vi "INIT_events_SD.vi"(2 "bounds":T2, 3 "references":T1) -> (0 "main cluster":T3={"Kinetics"=[], "Spectrum"=[], "Experiments groups"=[], "GRAPH EXPERIMENTAL DATA"=[], "error out"={"status"=FALSE, "code"=0, "source"=""}, "group"=0, "exp selected"=0, "# exp"=0, "kinetics plot names"=[], "spectra plot names"=[], "FromToWave"={"FromWave"=0.0, "ToWave"=0.0}, "Laser shutter task"="", "Accelerator task"="", "Motor task"="", "GRAPH EXPERIMENTAL DATA ref"=refnum, "timedelays"=[0.0, 0.0, 0.0, 0.0, 0.0, 0.0, 0.0, 0.06019061100911815, 0.0521779104562645, 0.045231877429679615, 0.03921051490799832, 0.033990728811568754, 0.029465811603150715, 0.025543260876973825, 0.02214288834180205, 0.01919518054014414, 0.016639877791965713, 0.014424742312398925, 0.012504490320209958, 0.010839866306230088, 0.009396840537117498, 0.008145913389103785, 0.00706151229029317, 0.006121468943269439, 0.005306566140927374, 0.004600144911132549, 0.003987763959109073, 0.0034569044455719407, 0.00299671406541447, 0.0025977851951783253, 0.0022519625739982996, 0.00195217658646366, 0.0016922987392150965, 0.0014670163768006634, 0.0012717240756200802, 0.0011024294957352762, 0.0009556717658856477, 0.0008284507332614981, 0.0007181656316962257, 0.0006225619144775864, 0.0005396851648867825, 0.00046784114226338394, 0.0004055611468220084, 0.0003515719951773376, 0.00030476999279031153, 0.00026419837125694315, 0.00022902772919263772, 0.0001985390768670671, 0.0001721091379728629, 0.00014919760805372974, 0.00012933610911736794], "wavelengths"=[0.0, 0.0, 0.0, 0.0, 0.0, 0.0, 0.0, 0.06019061100911815, 0.0521779104562645, 0.045231877429679615, 0.03921051490799832, 0.033990728811568754, 0.029465811603150715, 0.025543260876973825, 0.02214288834180205, 0.01919518054014414, 0.016639877791965713, 0.014424742312398925, 0.012504490320209958, 0.010839866306230088, 0.009396840537117498, 0.008145913389103785, 0.00706151229029317, 0.006121468943269439, 0.005306566140927374, 0.004600144911132549, 0.003987763959109073, 0.0034569044455719407, 0.00299671406541447, 0.0025977851951783253, 0.0022519625739982996, 0.00195217658646366, 0.0016922987392150965, 0.0014670163768006634, 0.0012717240756200802, 0.0011024294957352762, 0.0009556717658856477, 0.0008284507332614981, 0.0007181656316962257, 0.0006225619144775864, 0.0005396851648867825, 0.00046784114226338394, 0.0004055611468220084, 0.0003515719951773376, 0.00030476999279031153, 0.00026419837125694315, 0.00022902772919263772, 0.0001985390768670671, 0.0001721091379728629, 0.00014919760805372974, 0.00012933610911736794], "Experiment"=refnum, "Commentaires exp"=refnum, "FromToDelay"={"FromDelay"=0.0, "ToDelay"=0.0}}, 1 "Controls":T4)   [LabVIEW 2015]
uses:
  controls/Controls.ctl
  Classes/Experiment.lvclass
  controls/control-cluster.ctl
  Classes/Experiments_group.lvclass
  globalVarSD.vi
types:
  T1 = cluster{"Commentaires exp":refnum<vi>, "GRAPH EXPERIMENTAL DATA":refnum<vi>, "Experiment":refnum<vi>}
  T2 = cluster{"From Time":dbl, "To Time":dbl, "From Wave":dbl, "To Wave":dbl}
  T3 = typedef "control-cluster.ctl" = cluster{"Kinetics":cluster{"timedelay":dbl[], dbl[]}[], "Spectrum":cluster{"Unités abscisse":dbl[], dbl[]}[], "Experiments groups":refnum<class "Experiments_group.lvclass">[], "GRAPH EXPERIMENTAL DATA":dbl[][], "error out":errorcluster, "group":i32, "exp selected":i32, "# exp":i32, "kinetics plot names":string[], "spectra plot names":string[], "FromToWave":cluster{"FromWave":dbl, "ToWave":dbl}, "Laser shutter task":refnum<k21>, "Accelerator task":refnum<k21>, "Motor task":refnum<k21>, "GRAPH EXPERIMENTAL DATA ref":refnum<vi>, "timedelays":dbl[], "wavelengths":dbl[], "Experiment":refnum<vi>, "Commentaires exp":refnum<vi>, "FromToDelay":cluster{"FromDelay":dbl, "ToDelay":dbl}}
  T4 = typedef "Controls.ctl" = cluster{"Update graphs of exp":refnum<user-event>, "Reglage event":refnum<user-event>, "Stop event":refnum<user-event>, "notifier mesure out":refnum<notifier>, "notifier reglage out":refnum<notifier>, "Measure finished":refnum<user-event>, "control registration ref":refnum<event-registration>, "redraw event":refnum<user-event>, "Measure event":refnum<user-event>, "Mes, Reg, Stop Registration ref":refnum<event-registration>, "Laser shutter task":refnum<k21>, "error out":errorcluster, "Motor task":refnum<k21>, "Accelerator task":refnum<k21>, "Faraday Cup task":refnum<k21>, "Protection":refnum<event-registration>, "heater Alarm task":refnum<k21>, "Relay key task":refnum<k21>}
  T5 = cluster{"Heater alaram task":refnum<k21>, "Laser shutter task":refnum<k21>, "Motor task":refnum<k21>, "Accelerator shutter task":refnum<k21>, "Relay key task":refnum<k21>, "Faraday cup task":refnum<k21>}
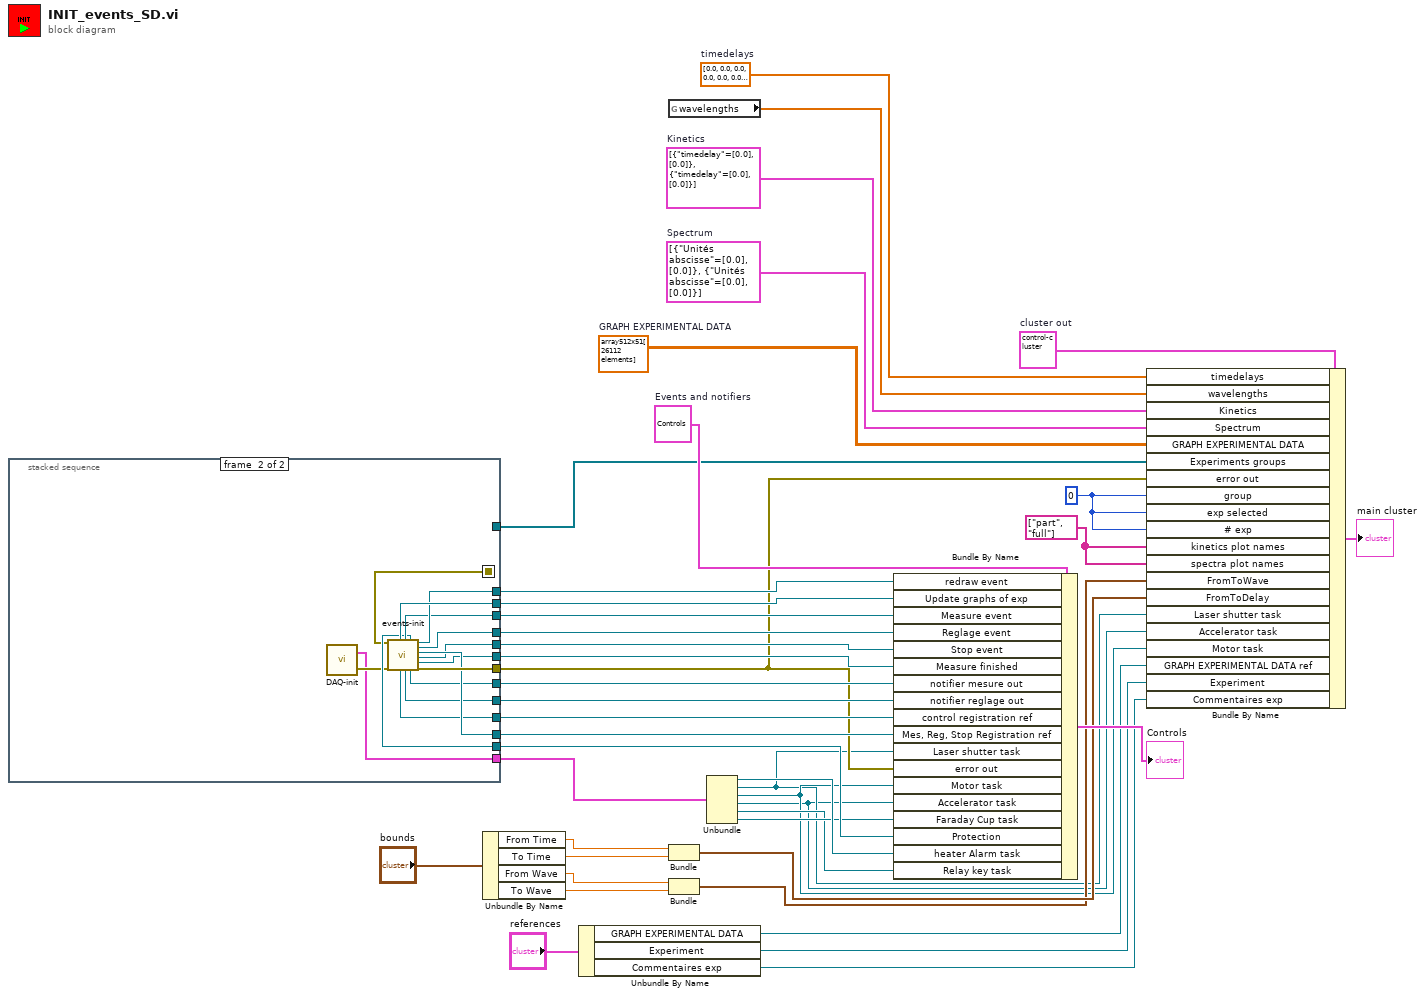
[diagram p0: block diagram]
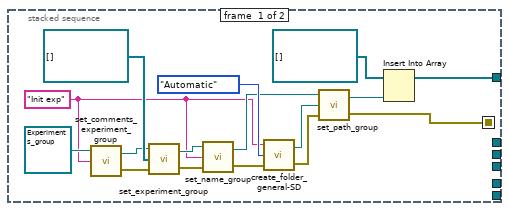
[diagram p2: hidden frame]
diagram:
  w18 = dbl[] [0.0, 0.0, 0.0, 0.0, 0.0, 0.0, 0.0, 0.06019061100911815, 0.0521779104562645, 0.045231877429679615, 0.03921051490799832, 0.033990728811568754, 0.029465811603150715, 0.025543260876973825, 0.02214288834180205, 0.01919518054014414, 0.016639877791965713, 0.014424742312398925, 0.012504490320209958, 0.010839866306230088, 0.009396840537117498, 0.008145913389103785, 0.00706151229029317, 0.006121468943269439, 0.005306566140927374, 0.004600144911132549, 0.003987763959109073, 0.0034569044455719407, 0.00299671406541447, 0.0025977851951783253, 0.0022519625739982996, 0.00195217658646366, 0.0016922987392150965, 0.0014670163768006634, 0.0012717240756200802, 0.0011024294957352762, 0.0009556717658856477, 0.0008284507332614981, 0.0007181656316962257, 0.0006225619144775864, 0.0005396851648867825, 0.00046784114226338394, 0.0004055611468220084, 0.0003515719951773376, 0.00030476999279031153, 0.00026419837125694315, 0.00022902772919263772, 0.0001985390768670671, 0.0001721091379728629, 0.00014919760805372974, 0.00012933610911736794]  # timedelays
  w27 = T3 {"Kinetics"=[], "Spectrum"=[], "Experiments groups"=[], "GRAPH EXPERIMENTAL DATA"=[], "error out"={"status"=FALSE, "code"=0, "source"=""}, "group"=0, "exp selected"=0, "# exp"=0, "kinetics plot names"=[], "spectra plot names"=[], "FromToWave"={"FromWave"=0.0, "ToWave"=0.0}, "Laser shutter task"="", "Accelerator task"="", "Motor task"="", "GRAPH EXPERIMENTAL DATA ref"=refnum, "timedelays"=[0.0, 0.0, 0.0, 0.0, 0.0, 0.0, 0.0, 0.06019061100911815, 0.0521779104562645, 0.045231877429679615, 0.03921051490799832, 0.033990728811568754, 0.029465811603150715, 0.025543260876973825, 0.02214288834180205, 0.01919518054014414, 0.016639877791965713, 0.014424742312398925, 0.012504490320209958, 0.010839866306230088, 0.009396840537117498, 0.008145913389103785, 0.00706151229029317, 0.006121468943269439, 0.005306566140927374, 0.004600144911132549, 0.003987763959109073, 0.0034569044455719407, 0.00299671406541447, 0.0025977851951783253, 0.0022519625739982996, 0.00195217658646366, 0.0016922987392150965, 0.0014670163768006634, 0.0012717240756200802, 0.0011024294957352762, 0.0009556717658856477, 0.0008284507332614981, 0.0007181656316962257, 0.0006225619144775864, 0.0005396851648867825, 0.00046784114226338394, 0.0004055611468220084, 0.0003515719951773376, 0.00030476999279031153, 0.00026419837125694315, 0.00022902772919263772, 0.0001985390768670671, 0.0001721091379728629, 0.00014919760805372974, 0.00012933610911736794], "wavelengths"=[0.0, 0.0, 0.0, 0.0, 0.0, 0.0, 0.0, 0.06019061100911815, 0.0521779104562645, 0.045231877429679615, 0.03921051490799832, 0.033990728811568754, 0.029465811603150715, 0.025543260876973825, 0.02214288834180205, 0.01919518054014414, 0.016639877791965713, 0.014424742312398925, 0.012504490320209958, 0.010839866306230088, 0.009396840537117498, 0.008145913389103785, 0.00706151229029317, 0.006121468943269439, 0.005306566140927374, 0.004600144911132549, 0.003987763959109073, 0.0034569044455719407, 0.00299671406541447, 0.0025977851951783253, 0.0022519625739982996, 0.00195217658646366, 0.0016922987392150965, 0.0014670163768006634, 0.0012717240756200802, 0.0011024294957352762, 0.0009556717658856477, 0.0008284507332614981, 0.0007181656316962257, 0.0006225619144775864, 0.0005396851648867825, 0.00046784114226338394, 0.0004055611468220084, 0.0003515719951773376, 0.00030476999279031153, 0.00026419837125694315, 0.00022902772919263772, 0.0001985390768670671, 0.0001721091379728629, 0.00014919760805372974, 0.00012933610911736794], "Experiment"=refnum, "Commentaires exp"=refnum, "FromToDelay"={"FromDelay"=0.0, "ToDelay"=0.0}}  # cluster out
  w26 = string[] ["part", "full"] ("kinetics plot names")
  w25 = 0 ("exp selected")
  w28 = dbl[][] array512x51[26112 elements]  # GRAPH EXPERIMENTAL DATA
  w30 = cluster{"timedelay":dbl[], dbl[]}[] [{"timedelay"=[0.0], [0.0]}, {"timedelay"=[0.0], [0.0]}]  # Kinetics
  w29 = cluster{"Unités abscisse":dbl[], dbl[]}[] [{"Unités abscisse"=[0.0], [0.0]}, {"Unités abscisse"=[0.0], [0.0]}]  # Spectrum
  w42 = T4 {"Update graphs of exp"=refnum, "Reglage event"=refnum, "Stop event"=refnum, "notifier mesure out"=refnum, "notifier reglage out"=refnum, "Measure finished"=refnum, "control registration ref"=refnum, "redraw event"=refnum, "Measure event"=refnum, "Mes, Reg, Stop Registration ref"=refnum, "Laser shutter task"="", "error out"={"status"=FALSE, "code"=0, "source"=""}, "Motor task"="", "Accelerator task"="", "Faraday Cup task"="", "Protection"=refnum, "heater Alarm task"="", "Relay key task"=""}  # Events and notifiers
  n1 = stacked-sequence {
    seq-local: [w49 _] -> [_ w61]
    tunnel: [_ w73] -> w22
    tunnel: [_ w72] -> w32
    tunnel: [_ w71] -> w38
    tunnel: [_ w70] -> w37
    tunnel: [_ w64] -> w33
    tunnel: [_ w69] -> w36
    tunnel: [_ w68] -> w41
    tunnel: [_ w67] -> w40
    tunnel: [_ w63] -> w39
    tunnel: [_ w66] -> w35
    tunnel: [_ w65] -> w34
    tunnel: [w43 _] -> w21
    tunnel: [_ w62] -> w19
    tunnel: [_ w59] -> w7
    frame #0 {
      w44 = "Init exp" ("Comments")
      n2 = call-dynamic "set_comments_experiment_group.vi"("Comments"=w44, "Experiments_group.lvclass in"=refnum<class "Experiments_group.lvclass"> refnum ("Experiments_group.lvclass")) -> ("error out"=w53:errorcluster, "Experiments_group.lvclass out"=w51:refnum<class "Experiments_group.lvclass">)  [unwired: 1 in]
      n3 = call-dynamic "set_experiment_group.vi"("error in (no error)"=w53, "Experiments"=refnum<class "Experiment.lvclass">[] [] ("Experiment array"), "Experiments_group.lvclass in"=w51) -> ("error out"=w48:errorcluster, "Experiments_group.lvclass out"=w46:refnum<class "Experiments_group.lvclass">)
      n4 = call-dynamic "set_name_group.vi"("error in (no error)"=w48, "Name"=w44, "Experiments_group.lvclass in"=w46) -> ("error out"=w47:errorcluster, "Experiments_group.lvclass out"=w45:refnum<class "Experiments_group.lvclass">)
      n5 = call "create_folder_general-SD.vi"("error in (no error)"=w47, "save Radio Buttons"=enum32{"Automatic", "User-def"}."Automatic", "Name"=w44) -> ("error out"=w55:errorcluster, "appended path"=w56:path)
      n6 = call-dynamic "set_path_group.vi"("error in (no error)"=w55, "Path"=w56, "Experiments_group.lvclass in"=w45) -> ("error out"=w49:errorcluster, "Experiments_group.lvclass out"=w50:refnum<class "Experiments_group.lvclass">)
      n7 = Insert Into Array(array=refnum<class "Experiments_group.lvclass">[] [] ("Experiments groups"), new element=w50) -> (w43:refnum<class "Experiments_group.lvclass">[])  [unwired: 1 in]
    }
    frame #1 {
      n8 = call "DAQ-init.vi"() -> ("sortie d'erreur"=w60:errorcluster, "cluster of DAQ tasks"=w59:T5)
      n9 = call "events-init.vi"("error out"=w61, "entrée d'erreur (pas d'erreur)"=w60) -> ("Update graphs of exp"=w68:refnum<user-event>, "Refnum d'abonnement à des événements 2"=w69:refnum<event-registration>, "Measure event"=w64:refnum<user-event>, "notifier out 2"=w71:refnum<notifier>, "Refnum d'abonnement à des événements"=w62:refnum<event-registration>, "notifier out"=w70:refnum<notifier>, "Événement utilisateur en sortie"=w65:refnum<user-event>, "Reglage event"=w67:refnum<user-event>, "Refnum d'abonnement à des événements 3"=w72:refnum<event-registration>, "Stop event"=w63:refnum<user-event>, "Measure finished"=w66:refnum<user-event>, "sortie d'erreur"=w73:errorcluster)  [unwired: 6 in]
    }
  }
  n10 = Unbundle By Name("bounds") -> ("From Time"=w15:dbl, "To Time"=w14:dbl, "From Wave"=w12:dbl, "To Wave"=w13:dbl)
  n11 = Unbundle By Name("references") -> ("GRAPH EXPERIMENTAL DATA"=w10:refnum<vi>, "Experiment"=w9:refnum<vi>, "Commentaires exp"=w8:refnum<vi>)
  n12 = global read "globalVarSD.vi" "wavelengths"() -> (w17:dbl[])
  n13 = Bundle("From Time"=w15, "To Time"=w14) -> (w24:cluster{"From Time":dbl, "To Time":dbl})  [unwired: 1 in]
  n14 = Bundle("From Wave"=w12, "To Wave"=w13) -> (w23:cluster{"From Wave":dbl, "To Wave":dbl})  [unwired: 1 in]
  n15 = Unbundle(w7) -> ("Heater alaram task"=w6:refnum<k21>, "Laser shutter task"=w2:refnum<k21>, "Motor task"=w3:refnum<k21>, "Accelerator shutter task"=w1:refnum<k21>, "Relay key task"=w4:refnum<k21>, "Faraday cup task"=w5:refnum<k21>)
  n16 = Bundle By Name(cluster=w42, "redraw event"=w34, "Update graphs of exp"=w41, "Measure event"=w33, "Reglage event"=w40, "Stop event"=w39, "Measure finished"=w35, "notifier mesure out"=w37, "notifier reglage out"=w38, "control registration ref"=w36, "Mes, Reg, Stop Registration ref"=w32, "Laser shutter task"=w2, "error out"=w22, "Motor task"=w3, "Accelerator task"=w1, "Faraday Cup task"=w5, "Protection"=w19, "heater Alarm task"=w6, "Relay key task"=w4) -> (→"Controls":T4)
  n17 = Bundle By Name(cluster=w27, "timedelays"=w18, "wavelengths"=w17, "Kinetics"=w30, "Spectrum"=w29, "GRAPH EXPERIMENTAL DATA"=w28, "Experiments groups"=w21, "error out"=w22, "group"=w25, "exp selected"=w25, "# exp"=w25, "kinetics plot names"=w26, "spectra plot names"=w26, "FromToWave"=w23, "FromToDelay"=w24, "Laser shutter task"=w2, "Accelerator task"=w1, "Motor task"=w3, "GRAPH EXPERIMENTAL DATA ref"=w10, "Experiment"=w9, "Commentaires exp"=w8) -> (→"main cluster":T3)
